vi "Project Image.vi"() -> ()   [LabVIEW 2012]
panel:
  in  "NonTearing? (True)":bool
  in  "stop":bool
  in  "Image Path 1":path=path "C:/Program Files/National Instruments/Vision/Examples/Images/Candy1.png"
  in  "Display Index":i32
  # "Instructions:\n1.  Verify that the Image Files exist at the paths specified in controls \"Image Path 1\"\n2.  Run the VI.\n3.  Move the image window so that half of it is in the 2nd display.\n4.  Notice that the image does not update on the 2nd display.\n\nExperiment with having NonTearing?\" ON or OFF (need to rerun VI) to see if the problem occurs."
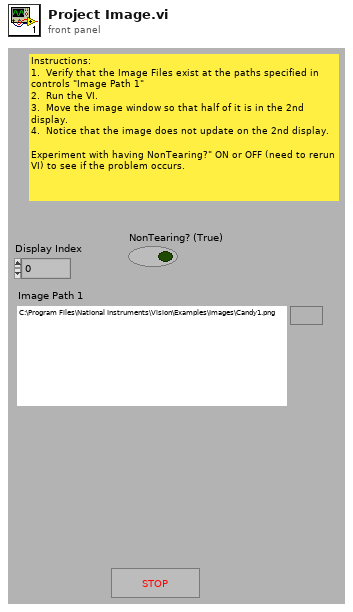
[diagram p1: front panel]
types:
  T1 = typedef "LVAllMonitorsDisplayTypeDef.ctl" = cluster{"Bounds":cluster{"Left":i16, "Top":i16, "Right":i16, "Bottom":i16}, "Depth":i16}[]
  T2 = cluster{"Bounds":cluster{"Left":i16, "Top":i16, "Right":i16, "Bottom":i16}, "Depth":i16}
  T3 = cluster{"Left":i16, "Top":i16, "Right":i16, "Bottom":i16}
  T4 = typedef "Image Type" = u32
  T5 = typedef "IMAQ Image.ctl" = refnum<image>
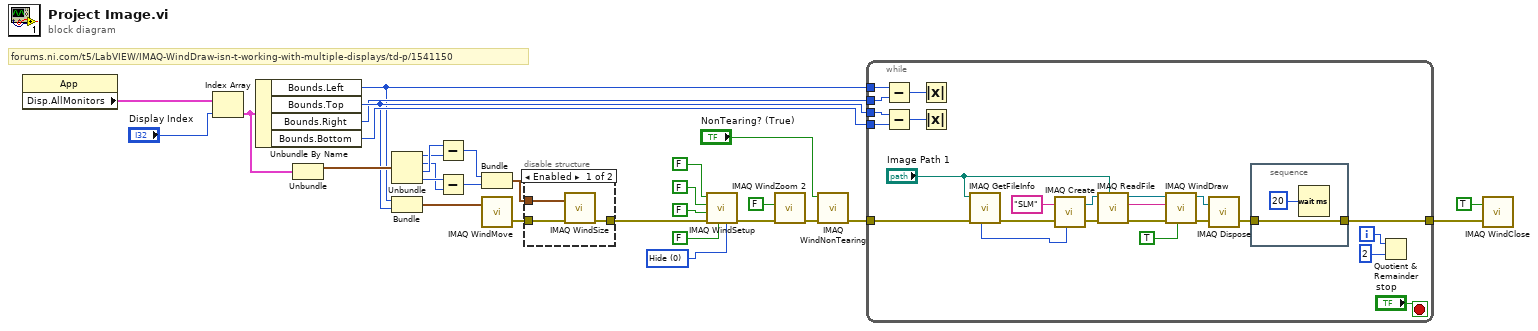
[diagram p0: block diagram]
diagram:
  w23 = 0 items=["Hide", "Show", "No change"] ("Scrollbars (No change)")
  # "forums.ni.com/t5/LabVIEW/IMAQ-WindDraw-isn-t-working-with-multiple-displays/td-p/1541150"
  n1 = property class="App"() -> ("Disp.AllMonitors"=w25:T1)  [unwired: 2 in, 2 out]
  n2 = Index Array(array=w25, index="Display Index") -> (element=w28:T2)
  n3 = Unbundle By Name(w28) -> ("Bounds.Left"=w2:i16, "Bounds.Top"=w4:i16, "Bounds.Right"=w3:i16, "Bounds.Bottom"=w5:i16)
  n4 = Unbundle(w28) -> ("Bounds"=w27:T3)  [unwired: 1 out]
  n5 = Unbundle(w27) -> ("Left"=w17:i16, "Top"=w15:i16, "Right"=w18:i16, "Bottom"=w16:i16)
  n6 = Bundle("Left"=w2, "Top"=w4) -> (w6:cluster{"Left":i16, "Top":i16})  [unwired: 1 in]
  n7 = Subtract(x=w18, y=w17) -> (x-y=w29:i16)
  n8 = Subtract(x=w16, y=w15) -> (x-y=w30:i16)
  n9 = Bundle(w29, w30) -> (w1:cluster{i16, i16})  [unwired: 1 in]
  n10 = call "IMAQ WindMove"("Coordinates (screen)"=w6) -> ("error out"=w21:errorcluster)  [unwired: 4 in, 1 out]
  n11 = disable-structure shown="Enabled" {
    disable-tunnel: w1 -> [w33 _]
    disable-tunnel: [w32 _] -> w14
    disable-tunnel: w21 -> [w31 _]
    frame Enabled {
      n12 = call "IMAQ WindSize"("error in (no error)"=w31, "Width & Height"=w33) -> ("error out"=w32:errorcluster)  [unwired: 4 in, 2 out]
    }
    frame Disabled {
    }
  }
  n13 = call "IMAQ WindSetup"("Scrollbars (No change)"=w23, "Window is floating? (No)"=FALSE, "error in (no error)"=w14, "Window has title bar? (Yes)"=FALSE, "Window can close? (Yes)"=FALSE, "Window can grow? (Yes)"=FALSE) -> ("error out"=w12:errorcluster)  [unwired: 5 in]
  n14 = call "IMAQ WindZoom 2"("error in (no error)"=w12, "Zoom to Fit? (False)"=FALSE ("Zoom to Fit? (T)")) -> ("error out"=w10:errorcluster)  [unwired: 6 in, 3 out]
  n15 = call "IMAQ WindNonTearing"("error in (no error)"=w10, "NonTearing? (True)"="NonTearing? (True)") -> ("error out"=w9:errorcluster)  [unwired: 8 in, 1 out]
  n16 = while {
    tunnel: w9 -> [w56]
    tunnel: [w48] -> w11
    tunnel: w5 -> [w47]
    tunnel: w4 -> [w46]
    tunnel: w3 -> [w45]
    tunnel: w2 -> [w44]
    i -> [w51]
    stop <- "stop" stop-if-true
    n17 = Subtract(x=w44, y=w45) -> (x-y=w43:i16)
    n18 = Subtract(x=w46, y=w47) -> (x-y=w42:i16)
    n19 = Absolute Value(x=w43) -> ()  [unwired: 1 out]
    n20 = Absolute Value(x=w42) -> ()  [unwired: 1 out]
    n21 = call "IMAQ GetFileInfo"("error in (no error)"=w56, "File Path"="Image Path 1") -> ("error out"=w41:errorcluster, "Image Type"=w40:T4)  [unwired: 3 in, 5 out]
    n22 = call "IMAQ Create"("Image Name"="SLM", "Image Type"=w40, "error in (no error)"=w41) -> ("New Image"=w36:T5, "error out"=w35:errorcluster)  [unwired: 2 in]
    n23 = call "IMAQ ReadFile"("File Path"="Image Path 1", "error in (no error)"=w35, "Image"=w36) -> ("error out"=w37:errorcluster, "File Type out"=w38:string, "Image Out"=w39:T5)  [unwired: 4 in, 2 out]
    n24 = call "IMAQ WindDraw"("Resize to Image Size? (Y)"=TRUE, "error in (no error)"=w37, "Title"=w38, "Image"=w39) -> ("error out"=w54:errorcluster, "Image Out (duplicate)"=w53:T5)  [unwired: 6 in]
    n25 = call "IMAQ Dispose"("Image"=w53, "error in (no error)"=w54) -> ("error out"=w49:errorcluster)  [unwired: 4 in]
    n26 = stacked-sequence {
      tunnel: w49 -> [w58]
      tunnel: [w58] -> w48
      frame #0 {
        n27 = Wait (ms)(milliseconds to wait=u32 20) -> ()  [unwired: 1 out]
      }
    }
    n28 = Quotient & Remainder(x=w51, y=2) -> ()  [unwired: 2 out]
  }
  n29 = call "IMAQ WindClose"("Close All Windows (False)"=TRUE, "error in (no error)"=w11) -> ()  [unwired: 4 in, 1 out]
